vi "Error Handler.vi"(7 "function":T2=enum."shm_open", 8 "error in (no error)":errorcluster, 11 "errno":T1) -> (0 "error out":errorcluster)   [LabVIEW 2013, in "Linux RT IPC.lvlib" / "Shared Memory.lvlib" / "Shared Memory.lvclass"]
doc: "This VI handles the errors returned by the Call Library Function Nodes used by this library. The C function errors are translated into LabVIEW errors to allow standard LabVIEW error handling."
uses:
  Shared Memory.lvclass
  Controls/functions.ctl
  <vilib>/NI/NI Linux RT Errno/Controls/Public/errno.ctl
  <vilib>/NI/NI Linux RT Errno/Linux Errno.lvlib
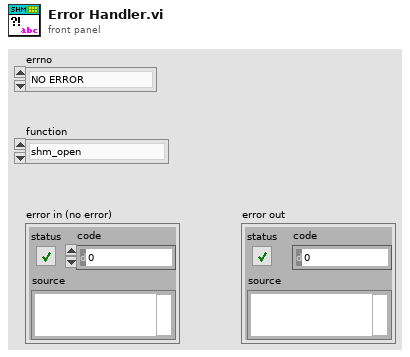
[diagram p1: front panel]
types:
  T1 = typedef "Linux Errno.lvlib/errno.ctl" = enum16{"NO ERROR", "EPERM", "ENOENT", "ESRCH", "EINTR", "EIO", "ENXIO", "E2BIG", "ENOEXEC", "EBADF", "ECHILD", "EAGAIN", "ENOMEM", "EACCES", "EFAULT", "ENOTBLK", "EBUSY", "EEXIST", "EXDEV", "ENODEV", "ENOTDIR", "EISDIR", "EINVAL", "ENFILE", "EMFILE", "ENOTTY", "ETXTBSY", "EFBIG", "ENOSPC", "ESPIPE", "EROFS", "EMLINK", "EPIPE", "EDOM", "ERANGE", "EDADLK", "ENAMETOOLONG", "ENOLCK", "ENOSYS", "ENOTEMPTY", "ELOOP", "EWOULDBLOCK", "ENOMSG", "EIDRM", "ECHRNG", "EL2NSYNC", "EL3HLT", "EL3RST", "ELNRNG", "EUNATCH", "ENOCSI", "EL2HLT", "EBADE", "EBADR", "EXFULL", "ENOANO", "EBADRQC", "EBADSLT", "EDEADLOCK", "EBFONT", "ENOSTR", "ENODATA", "ETIME", "ENOSR", "ENONET", "ENOPKG", "EREMOTE", "ENOLINK", "EADV", "ESRMNT", "ECOMM", "EPROTO", "EMULTIHOP", "EDOTDOT", "EBADMSG", "EOVERFLOW", "ENOTUNIQ", "EBADFD", "EREMCHG", "ELIBACC", "ELIBBAD", "ELIBSCN", "ELIBMAX", "ELIBEXEC", "ELISEQ", "ERESTART", "ESTRPIPE", "EUSERS", "ENOTSOCK", "EDESTADDRREQ", "EMSGSIZE", "EPROTOTYPE", "ENOPROTOOPT", "EPROTONOSUPPORT", "ESOCKTNOSUPPORT", "EOPNOTSUPP", "EPFNOSUPPORT", "EAFNOSUPPORT", "EADDRINUSE", "EADDRNOTAVAIL", "ENETDOWN", "ENETUNREACH", "ENETRESET", "ECONNABORTED", "ECONNRESET", "ENOBUFS", "EISCONN", "ENOTCONN", "ESHUTDOWN", "ETOOMANYREFS", "ETIMEDOUT", "ECONNREFUSED", "EHOSTDOWN", "EHOSTUNREACH", "EALREADY", "EINPROGRESS", "ESTALE", "EUCLEAN", "ENOTNAM", "ENAVAIL", "EISNAM", "EREMOTEIO", "EDQUOT", "ENOMEDIUM", "EMEDIUMTYPE", "ECANCELED", "ENOKEY", "EKEYEXPIRED", "EKEYREVOKED", "EKEYREJECTED", "EOWNERDEAD", "ENOTRECOVERABLE", "ERFKILL", "EHWPOISON", "UNDEFINED"}
  T2 = typedef "Linux RT IPC.lvlib/Shared Memory.lvlib/Shared Memory.lvclass/functions.ctl" = enum16{"unspecified", "shm_open", "ftruncate", "mmap", "munmap", "close", "shm_unlink", "fstat"}
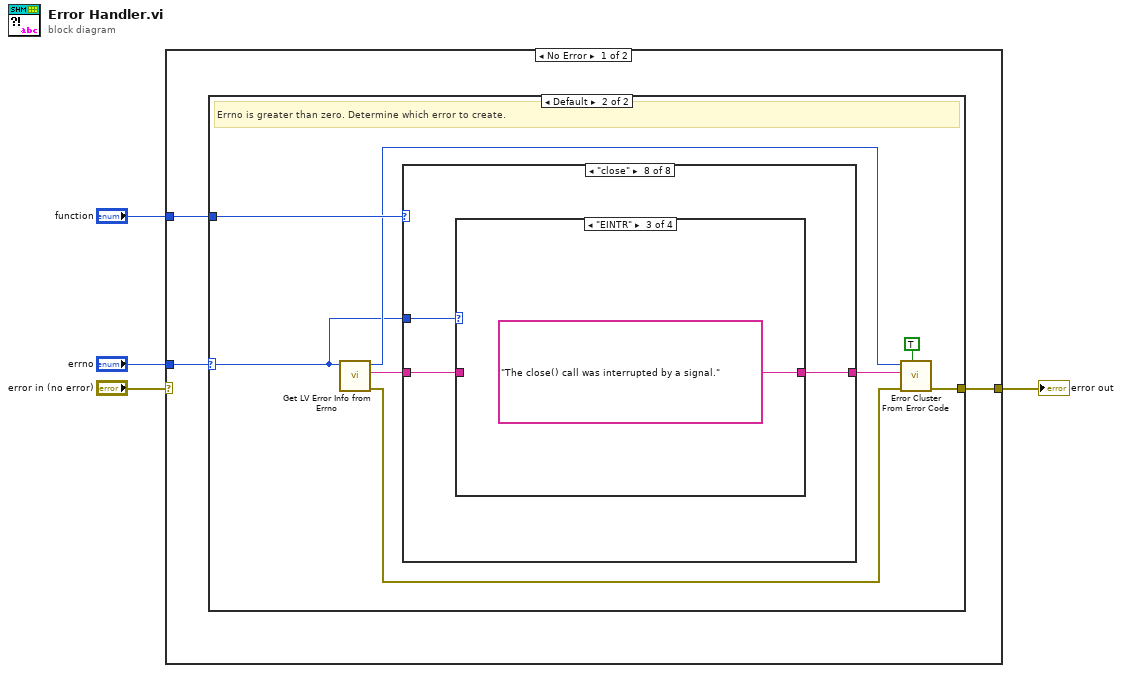
[diagram p0: block diagram]
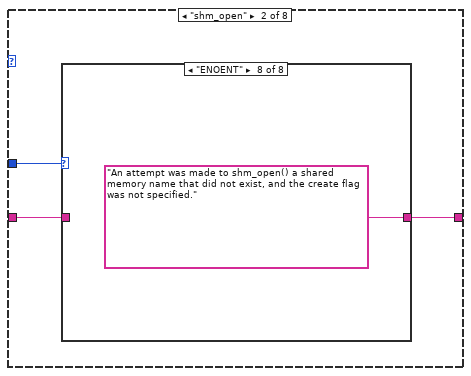
[diagram p4: hidden frame]
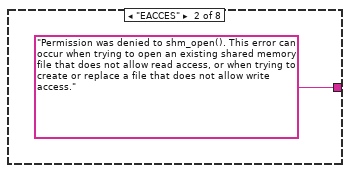
[diagram p6: hidden frame]
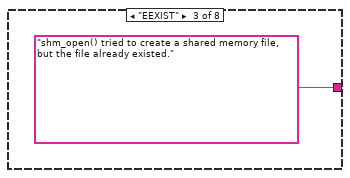
[diagram p7: hidden frame]
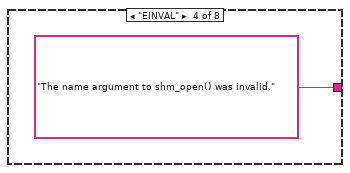
[diagram p8: hidden frame]
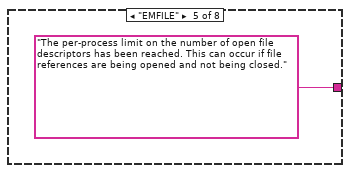
[diagram p9: hidden frame]
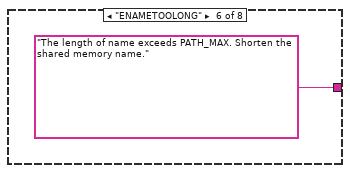
[diagram p10: hidden frame]
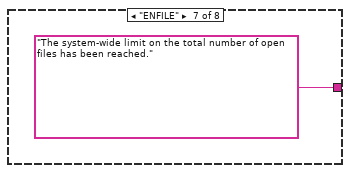
[diagram p11: hidden frame]
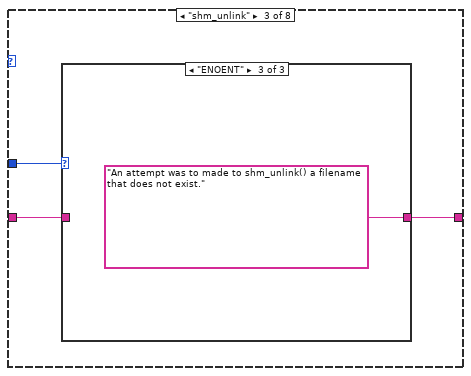
[diagram p12: hidden frame]
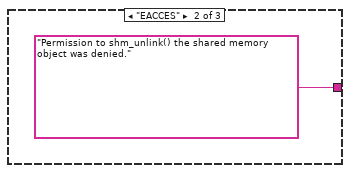
[diagram p14: hidden frame]
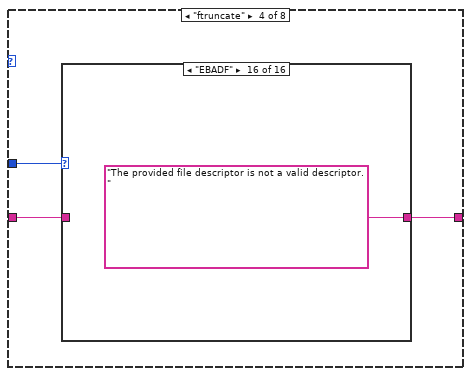
[diagram p15: hidden frame]
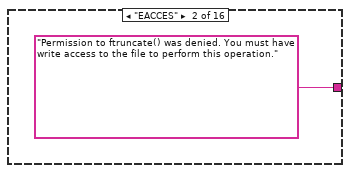
[diagram p17: hidden frame]
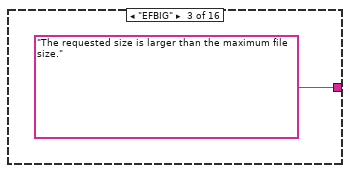
[diagram p18: hidden frame]
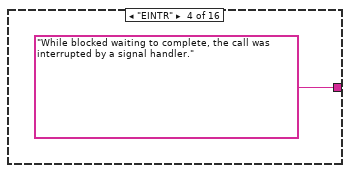
[diagram p19: hidden frame]
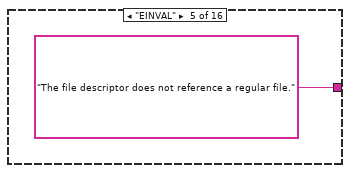
[diagram p20: hidden frame]
diagram:
  n1 = case shown="No Error" "error in (no error)" {
    selector: "error in (no error)" -> [_ w93]
    tunnel: [w7 w93] -> w3
    tunnel: "function" -> [w6 _]
    tunnel: "errno" -> [w5 _]
    frame No Error {
      n2 = case shown="Default" w5 {
        selector: w5 -> [_ w8]
        tunnel: [_ w15] -> w7
        tunnel: w6 -> [_ w13]
        frame "NO ERROR" {
          # "Errno is zero. No error occurred."
        }
        frame Default {
          # "Errno is greater than zero. Determine which error to create."
          n3 = call <vilib>:"Get LV Error Info from Errno.vi"("errno"=w8) -> ("error out"=w9:errorcluster, "error description"=w10:string, "error code"=w11:i32)  [unwired: 8 in]
          n4 = case shown="\"close\"" w13 {
            tunnel: w8 -> [_ w19 w30 w36 w55 w69 w75 w88]
            tunnel: [w16 w18 w29 w35 w54 w68 w74 w87] -> w12
            tunnel: w10 -> [w16 w17 w28 w34 w53 w67 w73 w86]
            frame "unspecified", Default {
              # "No specific function was specified, so use generic error description."
            }
            frame "shm_open" {
              n5 = case shown="\"ENOENT\"" w19 {
                tunnel: [w20 "Permission was denied to shm_open(). This error can occur when trying to open an existing shared memory file that does not allow read access, or when trying to create or replace a file that does not allow write access." "shm_open() tried to create a shared memory file, but the file already existed." "The name argument to shm_open() was invalid." "The per-process limit on the number of open file descriptors has been reached. This can occur if file references are being opened and not being closed." "The length of name exceeds PATH_MAX. Shorten the shared memory name." "The system-wide limit on the total number of open files has been reached." "An attempt was made to shm_open() a shared memory name that did not exist, and the create flag was not specified."] -> w18
                tunnel: w17 -> [w20 _ _ _ _ _ _ _]
                frame "NO ERROR", Default {
                }
                frame "EACCES" {
                }
                frame "EEXIST" {
                }
                frame "EINVAL" {
                }
                frame "EMFILE" {
                }
                frame "ENAMETOOLONG" {
                }
                frame "ENFILE" {
                }
                frame "ENOENT" {
                }
              }
            }
            frame "shm_unlink" {
              n6 = case shown="\"ENOENT\"" w30 {
                tunnel: [w31 "Permission to shm_unlink() the shared memory object was denied." "An attempt was to made to shm_unlink() a filename that does not exist."] -> w29
                tunnel: w28 -> [w31 _ _]
                frame "NO ERROR", Default {
                }
                frame "EACCES" {
                }
                frame "ENOENT" {
                }
              }
            }
            frame "ftruncate" {
              n7 = case shown="\"EBADF\"" w36 {
                tunnel: [w37 "Permission to ftruncate() was denied. You must have write access to the file to perform this operation." "The requested size is larger than the maximum file size." "While blocked waiting to complete, the call was interrupted by a signal handler." "The file descriptor does not reference a regular file." "An I/O error occurred updating the inode." "The named file is a directory." "Too many symbolic links were encountered in translating the pathname." "The length of name exceeds PATH_MAX." "The system-wide limit on the total number of open files has been reached." "The named file does not exist." "A component of the path prefix is not a directory." "The underlying file system does not support extending a file beyond its current size." "The named file resides on a read-only file system." "The file is a pure procedure (shared text) file that is being executed." "The provided file descriptor is not a valid descriptor."] -> w35
                tunnel: w34 -> [w37 _ _ _ _ _ _ _ _ _ _ _ _ _ _ _]
                frame "NO ERROR", Default {
                }
                frame "EACCES" {
                }
                frame "EFBIG" {
                }
                frame "EINTR" {
                }
                frame "EINVAL" {
                }
                frame "EIO" {
                }
                frame "EISDIR" {
                }
                frame "ELOOP" {
                }
                frame "ENAMETOOLONG" {
                }
                frame "ENFILE" {
                }
                frame "ENOENT" {
                }
                frame "ENOTDIR" {
                }
                frame "EPERM" {
                }
                frame "EROFS" {
                }
                frame "ETXTBSY" {
                }
                frame "EBADF" {
                }
              }
            }
            frame "mmap" {
              n8 = case shown="\"EACCES\"" w55 {
                tunnel: [w56 "File access/permission error. The cause of the error is due to one of the following reasons:\n1. A file descriptor refers to a non-regular file.\n2. A file mapping was requested, but the file descriptor is not open for reading.\n3. Mapping for a shared process was requested and and write access is requested, but the file descriptor is not open in read/write mode.\n4. Write access is requested, but the file is append-only." "The file has been locked, or too much memory has been locked." "The file descriptor is not a valid file descriptor (and MAP_ANONYMOUS was not set)." "An input parameter to mmap() was invalid. Possible issues are:\n1. The requested length was zero (nothing to map).\n2. The offset was not a multiple of the system's page size (and therefore wasn't lined up on a page boundary).\n3. flags contained neither MAP_PRIVATE or MAP_SHARED, or contained both of these values." "The system-wide limit on the total number of open files has been reached." "The underlying filesystem of the specified file does not support memory mapping." "No memory is available. The process's maximum number of mappings could have been exceeded." "The prot argument asks for PROT_EXEC but the mapped area belongs to a file on a filesystem that was mounted no-exec. Or, the operation was prevented by a file seal." "MAP_DENYWRITE was set but the object specified by fd is open for writing." "On 32-bit architecture together with the large file extension (i.e., using 64-bit off_t): the number of pages used for length plus number of pages used for offset would overflow unsigned long (32 bits)."] -> w54
                tunnel: w53 -> [w56 _ _ _ _ _ _ _ _ _ _]
                frame "NO ERROR", Default {
                }
                frame "EACCES" {
                }
                frame "EAGAIN" {
                }
                frame "EBADF" {
                }
                frame "EINVAL" {
                }
                frame "ENFILE" {
                }
                frame "ENODEV" {
                }
                frame "ENOMEM" {
                }
                frame "EPERM" {
                }
                frame "ETXTBSY" {
                }
                frame "EOVERFLOW" {
                }
              }
            }
            frame "munmap" {
              n9 = case shown="\"NO ERROR\", Default" w69 {
                tunnel: [w70 "An input parameter to munmap() was invalid. Possible issues are:\nLength of memory to unmap was zero." "No memory is available. This error can occur for munmap() if unmapping is attempted while the same region in memory is being mapped concurrently."] -> w68
                tunnel: w67 -> [w70 _ _]
                frame "NO ERROR", Default {
                }
                frame "EINVAL" {
                }
                frame "ENOMEM" {
                }
              }
            }
            frame "fstat" {
              n10 = case shown="\"NO ERROR\", Default" w75 {
                tunnel: [w76 "Search permission is denied for one of the directories in the path prefix of path." "File descriptor is invalid." "Bad address." "Too many symbolic links encountered while traversing the path." "Provided path is too long." "A component of path does not exist, or path is an empty string." "Out of memory (i.e., kernel memory)." "A component of the path prefix of path is not a directory." "Path or fd refers to a file whose size, inode number, or number of blocks cannot be represented in, respectively, the types off_t, ino_t, or blkcnt_t. This error can occur when, for example, an application compiled on a 32-bit platform without -D_FILE_OFFSET_BITS=64 calls stat() on a file whose size exceeds (1<<31)-1 bytes."] -> w74
                tunnel: w73 -> [w76 _ _ _ _ _ _ _ _ _]
                frame "NO ERROR", Default {
                }
                frame "EACCES" {
                }
                frame "EBADF" {
                }
                frame "EFAULT" {
                }
                frame "ELOOP" {
                }
                frame "ENAMETOOLONG" {
                }
                frame "ENOENT" {
                }
                frame "ENOMEM" {
                }
                frame "ENOTDIR" {
                }
                frame "EOVERFLOW" {
                }
              }
            }
            frame "close" {
              n11 = case shown="\"EINTR\"" w88 {
                tunnel: [w89 "The provided file descriptor is not valid." "The close() call was interrupted by a signal." "An I/O error occurred."] -> w87
                tunnel: w86 -> [w89 _ _ _]
                frame "NO ERROR", Default {
                }
                frame "EBADF" {
                }
                frame "EINTR" {
                }
                frame "EIO" {
                }
              }
            }
          }
          n12 = call <vilib>:"Error Cluster From Error Code.vi"("show call chain? (False)"=TRUE, "error in (no error)"=w9, "error message (\"\")"=w12, "error code (0)"=w11) -> ("error out"=w15:errorcluster)  [unwired: 5 in]
        }
      }
    }
    frame Error {
      # "Error already exists. Pass through."
    }
  }
  "error out" <- w3
